vi "Teleop.vi"(10 "Match Info":T1={"Autonomous Elapsed Seconds"=0.0, "TeleOp Elapsed Seconds"=0.0, "Disabled Elapsed Seconds"=0.0, "Visited Autonomous"=FALSE, "Visited TeleOp"=FALSE, "Visited Disabled"=FALSE, "Autonomous Settings"={"Autonomous Style"=enum."Independent", "VI Refnum"=refnum}}, 11 "Call Context":T2) -> ()   [LabVIEW 2013]
doc: "This VI is called for each TeleOp packet received from the DS where the robot is not disabled. It is often used to read from the joysticks and update I/O or to update setpoints for timed control loops. It should complete and return within 20 milliseconds or it may miss DS packets."
uses:
  <vilib>/Rock Robotics/WPI/DriverStation/WPI_DriverStationDerivedRobotMode.ctl
  <vilib>/Rock Robotics/WPI/DriverStation/WPI_DriverStationMatch Info.ctl
  <vilib>/Rock Robotics/WPI/Relay/WPI_RelayValue.ctl
  Robot Global Data.vi
  <vilib>/Rock Robotics/WPI/RobotDrive/WPI_RobotDriveMecanumDrive_Cartesian.vi
  <vilib>/Rock Robotics/WPI/Joystick/WPI_JoystickGetSetRefNum.vi
  <vilib>/functionblocks/Edge Detection/Edge Detect/Edge Detect.vi
  <vilib>/Rock Robotics/WPI/RobotDrive/WPI_RobotDriveGetSetRefNum.vi
  <vilib>/functionblocks/FB Core/FB Core.xnode
  <vilib>/functionblocks/NI_FunctionBlock Libraries.lvlib
panel:
  in  "percent":dbl
  out "Loader Up":bool
  out "Right Trigger":bool
  out "Left Trigger":bool
  out "Loader Out":bool
  out "Ejector":bool
  out "Trigger":bool
  out "1 Cylinder":bool
  out "2 Cylinder":bool
  out "3 Cylinder":bool
  out "Motor Values":dbl[](array[numeric])
  out "Gyro Mode?":bool
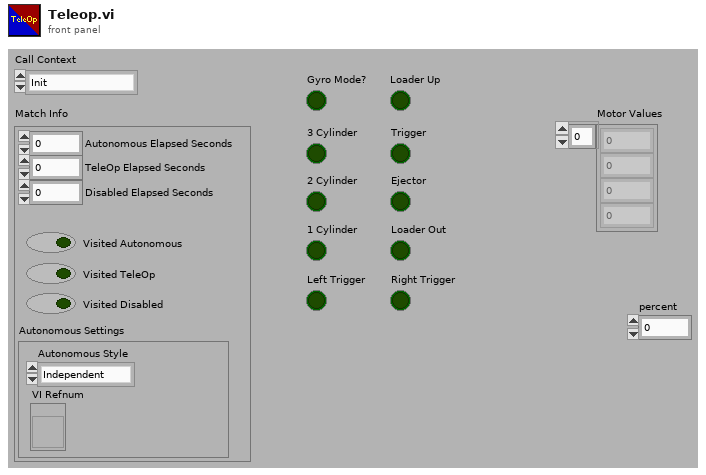
[diagram p1: front panel]
types:
  T1 = typedef "WPI_DriverStationMatch Info.ctl" = cluster{"Autonomous Elapsed Seconds":dbl, "TeleOp Elapsed Seconds":dbl, "Disabled Elapsed Seconds":dbl, "Visited Autonomous":bool, "Visited TeleOp":bool, "Visited Disabled":bool, "Autonomous Settings":cluster{"Autonomous Style":enum16{"Iterative", "Independent"}, "VI Refnum":refnum<vi>}}
  T2 = typedef "WPI_DriverStationDerivedRobotMode.ctl" = enum16{"Init", "Execute", "Stop"}
  T3 = typedef "WPI_RelayValue.ctl" = enum16{"Off", "On", "Forward", "Reverse"}
  T4 = typedef "WPI_MotorControlDeviceRef.ctl" = cluster{"DeviceStatus":errorcluster, "Type":enum16{"PWM", "CAN"}, "PWM":cluster{"Digital Module":T5, "PWM Channel":T6, "DeadBand":T7}, "CAN":cluster{"Device Number":u8, "Control Mode":T8, "Semaphore":T9, "Max Vout":dbl}, "Invert":bool, "TransformRef":T10, "InvTransformRef":T10}
  T5 = typedef "FPGA_TypedefDigitalModule.ctl" = enum16{"Digital Module 1", "Digital Module 2"}
  T6 = typedef "FPGA_DIOPWMChannel.ctl" = enum8{"PWM 1", "PWM 2", "PWM 3", "PWM 4", "PWM 5", "PWM 6", "PWM 7", "PWM 8", "PWM 9", "PWM 10", "Invalid"}
  T7 = typedef "WPI_PWMDeadband.ctl" = cluster{"Name":string, "maxPositivePwm":i32, "minPositivePwm":i32, "centerPwm":i32, "maxNegativePwm":i32, "minNegativePwm":i32, "angularRange":u16}
  T8 = typedef "WPI_CANJaguar_ControlMode.ctl" = enum8{"Percent VBus", "Current", "Speed", "Position", "Voltage"}
  T9 = typedef "Semaphore RefNum" = refnum<k1>
  T10 = typedef "WPI_PWMTransform_ConPane.ctl" = refnum<vi>
  T11 = typedef "WPI_JoystickDevRef.ctl" = cluster{"Device":T12}
  T12 = typedef "WPI_JoystickDeviceEnum.ctl" = enum16{"USB 1", "USB 2", "USB 3", "USB 4", "Kinect 1", "Kinect 2"}
  T13 = typedef "WPI_JoystickButtonState.ctl" = cluster{"Button 1":bool, "Button 2":bool, "Button 3":bool, "Button 4":bool, "Button 5":bool, "Button 6":bool, "Button 7":bool, "Button 8":bool, "Button 9":bool, "Button 10":bool, "Button 11":bool, "Button 12":bool}
  T14 = cluster{"axis 1 (x)":dbl, "axis 2 (y)":dbl, "axis 3 (throttle)":dbl, "axis 4":dbl, "axis 5":dbl, "axis 6":dbl}
  T15 = typedef "WPI_RelayDevRef.ctl" = cluster{"DevStatus":errorcluster, "Relay Channel":T16, "Digital Module":T5, "Relay Direction":T17}
  T16 = typedef "FPGA_DIORelayChannel.ctl" = enum8{"Relay 1", "Relay 2", "Relay 3", "Relay 4", "Relay 5", "Relay 6", "Relay 7", "Relay 8", "Invalid"}
  T17 = typedef "WPI_RelayDirection.ctl" = enum16{"Both directions", "Forward only", "Reverse only"}
  T18 = typedef "WPI_RobotDriveDevRef.ctl" = cluster{"DevStatus":errorcluster, "Motors[]":T4[], "Square Inputs":bool, "Max Output":dbl, "Isochronous":bool}
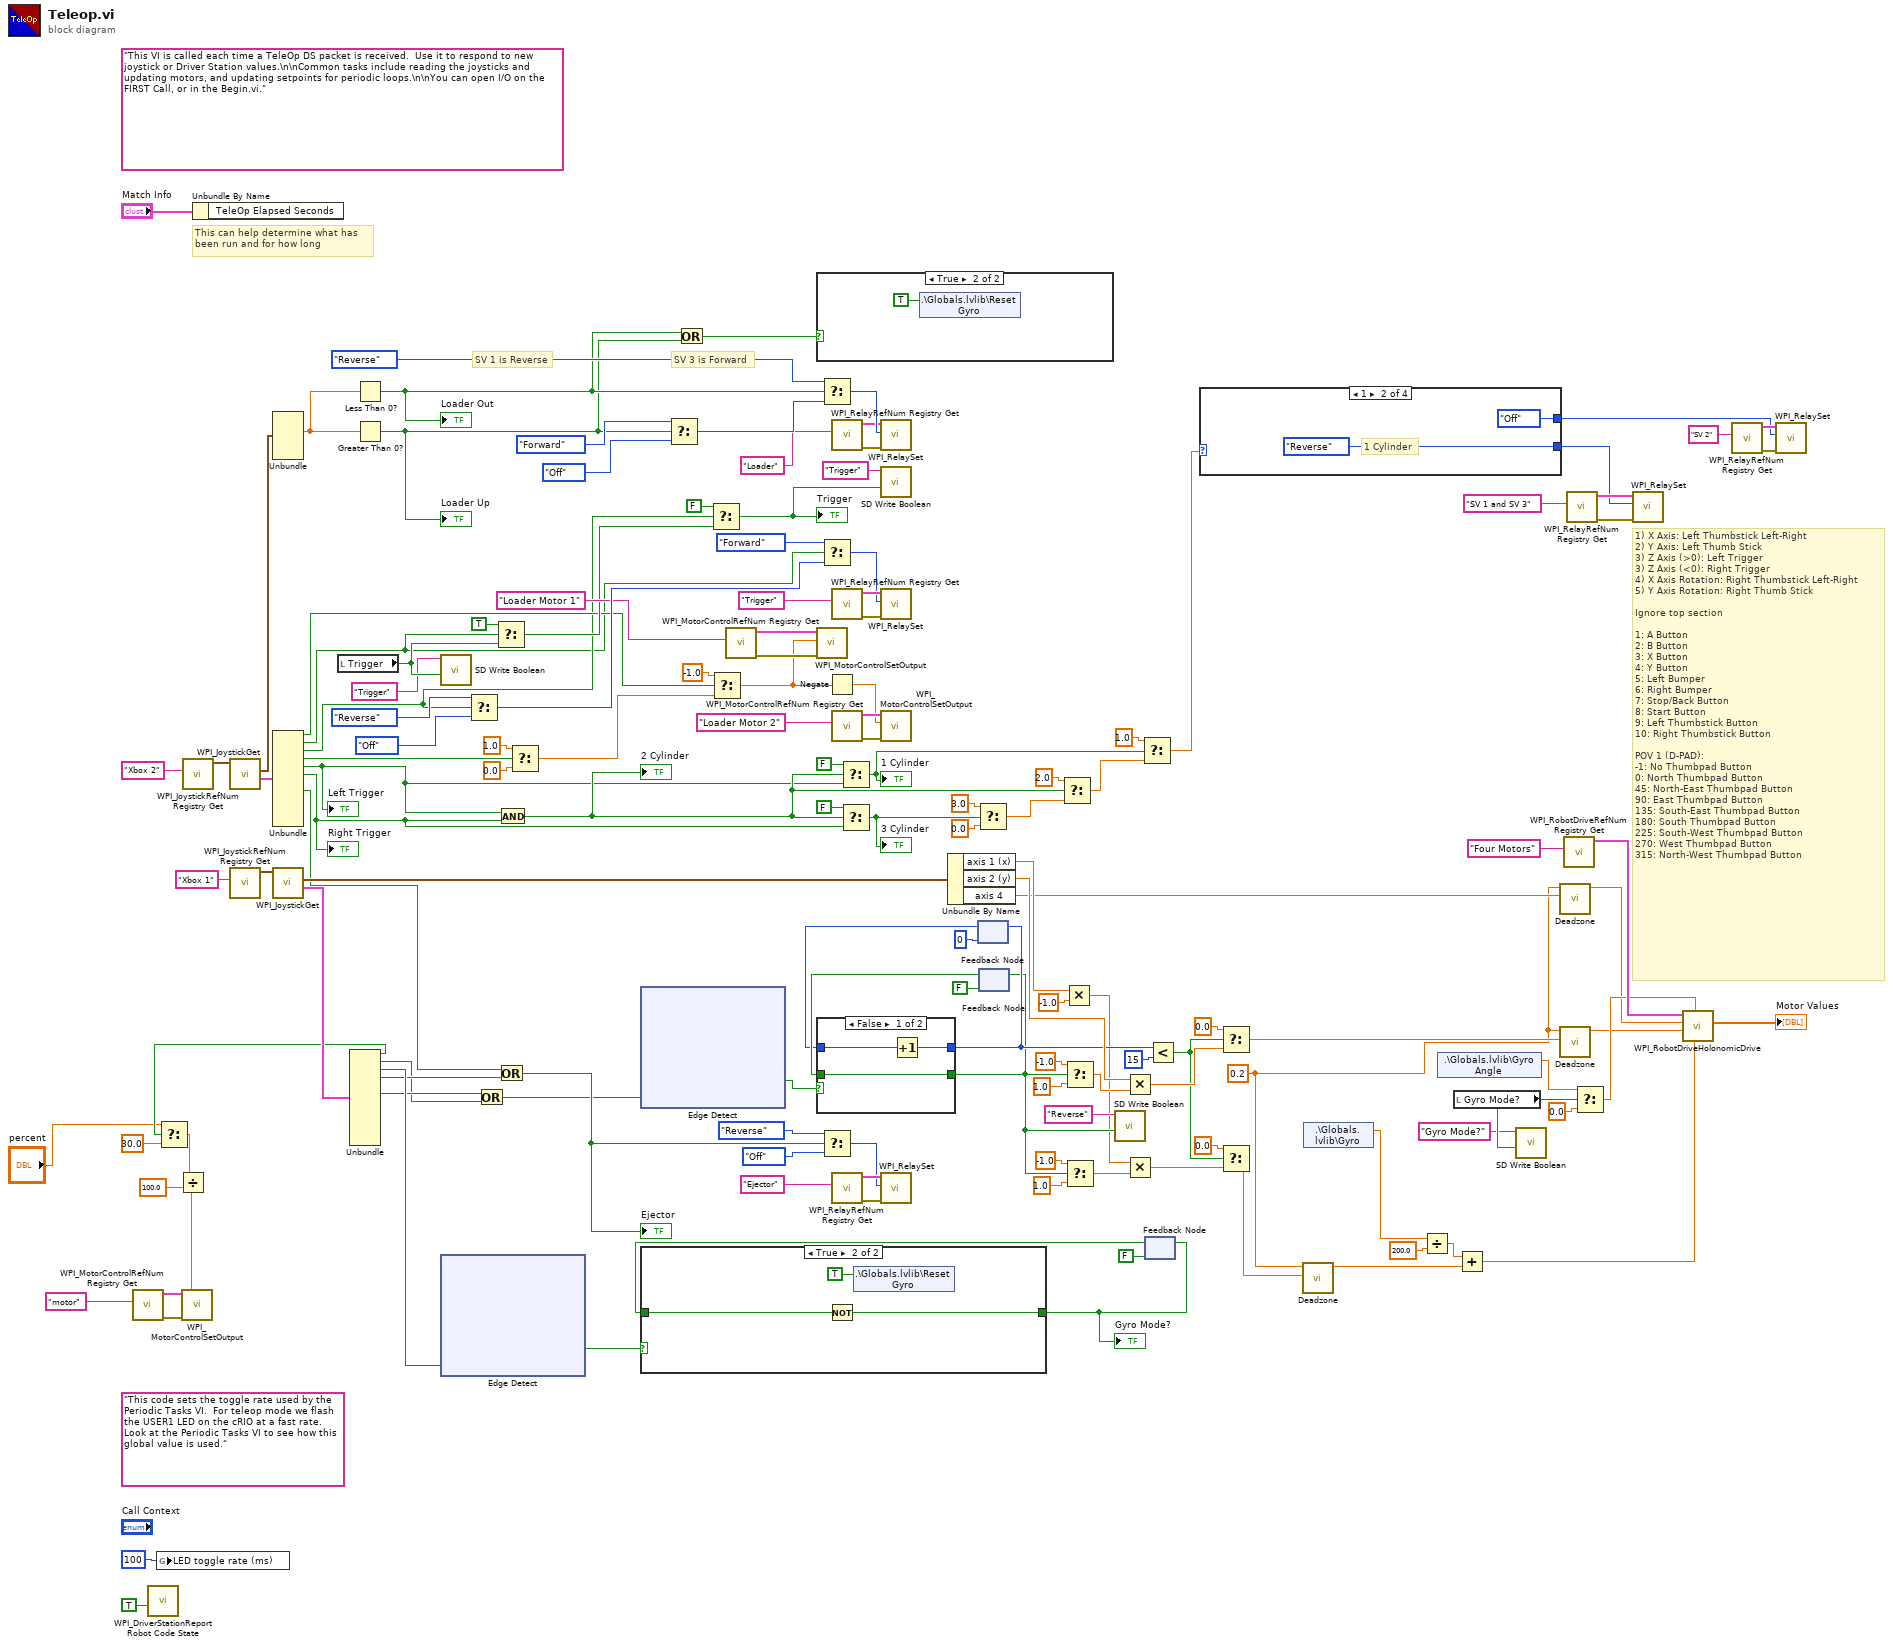
[diagram p0: block diagram]
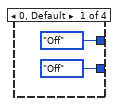
[diagram p3: hidden frame]
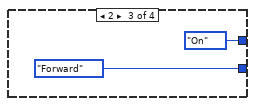
[diagram p4: hidden frame]
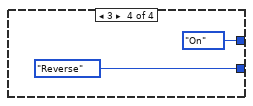
[diagram p5: hidden frame]
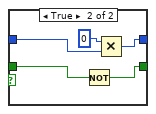
[diagram p6: hidden frame]
diagram:
  w19 = 0.2 ("Deadzone")
  (unwired) "This code sets the toggle rate used by the Periodic Tasks VI.  For teleop mode we flash the USER1 LED on the cRIO at a fast rate.  Look at the Periodic Tasks VI to see how this global value is used."
  (unwired) "This VI is called each time a TeleOp DS packet is received.  Use it to respond to new joystick or Driver Station values.\n\nCommon tasks include reading the joysticks and updating motors, and updating setpoints for periodic loops.\n\nYou can open I/O on the FIRST Call, or in the Begin.vi."
  # "SV 3 is Forward"
  # "SV 1 is Reverse"
  # "1) X Axis: Left Thumbstick Left-Right\n2) Y Axis: Left Thumb Stick\n3) Z Axis (>0): Left Trigger\n3) Z Axis (<0): Right Trigger\n4) X Axis Rotation: Right Thumbstick Left-Right\n5) Y Axis Rotation: Right Thumb Stick\n\nIgnore top section\n\n1: A Button\n2: B Button\n3: X Button\n4: Y Button\n5: Left Bumper\n6: Right Bumper\n7: Stop/Back Button\n8: Start Button\n9: Left Thumbstick Button\n10: Right Thumbstick Button\n\nPOV 1 (D-PAD):\n-1: No Thumbpad Button\n0: North Thumbpad Button\n45: North-East Thumbpad Button\n90: East Thumbpad Button\n135: South-East Thumbpad Button\n180: South Thumbpad Button\n225: South-West Thumbpad Button\n270: West Thumbpad Button\n315: North-West Thumbpad Button"
  # "This can help determine what has\nbeen run and for how long"
  n1 = call <vilib>:"WPI_MotorControlRefNum Registry Get.vi"("refnum name"="motor") -> ("error out"=w7:errorcluster, "MotorControlDevRef"=w8:T4)  [unwired: 9 in]
  n2 = call <vilib>:"WPI_DriverStationReport Robot Code State.vi"("TeleOp"=TRUE ("Autonomous")) -> ()  [unwired: 10 in, 1 out]
  n3 = global write "Robot Global Data.vi" "LED toggle rate (ms)"(u32 100 ("LED ms toggle rate")) -> ()
  n4 = call <vilib>:"WPI_JoystickRefNum Registry Get.vi"("refnum name"="Xbox 2") -> ("JoystickDevRef"=w112:T11)  [unwired: 1 in, 9 out]
  n5 = Unbundle By Name("Match Info") -> ()  [unwired: 1 out]
  n6 = call <vilib>:"WPI_JoystickGet.vi"("JoystickDevRef"=w112) -> ("Buttons"=w110:T13, "Axes"=w109:T14)  [unwired: 1 in, 4 out]
  n7 = call <vilib>:"WPI_JoystickRefNum Registry Get.vi"("refnum name"="Xbox 1") -> ("JoystickDevRef"=w143:T11)  [unwired: 1 in, 9 out]
  n8 = Unbundle(w109) -> ("axis 3 (throttle)"=w44:dbl)  [unwired: 5 out]
  n9 = Unbundle(w110) -> ("Button 1"=w32:bool, "Button 2"=w29:bool, "Button 3"=w30:bool, "Button 4"=w31:bool, "Button 5"=w45:bool, "Button 6"=w46:bool, "Button 8"=w35:bool)  [unwired: 5 out]
  "Left Trigger" <- w45
  "Right Trigger" <- w46
  n10 = call <vilib>:"WPI_JoystickGet.vi"("JoystickDevRef"=w143) -> ("Buttons"=w135:T13, "Axes"=w140:T14)  [unwired: 1 in, 4 out]
  n11 = local read "Trigger"() -> (w48:bool)
  n12 = Unbundle(w135) -> ("Button 1"=w6:bool, "Button 2"=w21:bool, "Button 3"=w49:bool, "Button 4"=w33:bool, "Button 6"=w22:bool)  [unwired: 7 out]
  n13 = Select(t="percent", s=w6, f=30.0) -> (s? t:f=w4:dbl)
  n14 = Divide(x=w4, y=100.0) -> (x/y=w2:dbl)
  n15 = call <vilib>:"WPI_MotorControlSetOutput.vi"("error in (no error)"=w7, "Output"=w2, "MotorControlDevRef"=w8) -> ()  [unwired: 6 in, 3 out]
  n16 = Less Than 0?(x=w44) -> (x < 0?=w17:bool)
  "Loader Out" <- w17
  n17 = Greater Than 0?(x=w44) -> (x > 0?=w16:bool)
  "Loader Up" <- w16
  n18 = call <vilib>:"SD Write Boolean.vi"("Boolean"=w48, "Name"="Trigger") -> ()  [unwired: 8 in, 2 out]
  n19 = xnode "Edge Detect"("input 1"=w49) -> ("output"=w53:bool)  [unwired: 2 in, 1 out]
  n20 = Select(t=WPI_RelayValue."Reverse" ("RelayValue"), s=w30, f=WPI_RelayValue."Off") -> (s? t:f=w91:T3)
  n21 = Or(x=w22, y=w21) -> (x .or. y?=w20:bool)
  n22 = Select(t=TRUE, s=w29, f=w48) -> (s? t:f=w60:bool)
  n23 = Or(x=w35, y=w33) -> (x .or. y?=w34:bool)
  "Ejector" <- w34
  n24 = And(x=w45, y=w46) -> (x .and. y?=w70:bool)
  "2 Cylinder" <- w70
  n25 = Select(t=1.0, s=w31, f=0.0) -> (s? t:f=w58:dbl)
  n26 = xnode "Edge Detect"("input 1"=w20) -> ("output"=w120:bool)  [unwired: 2 in, 1 out]
  n27 = Select(t=WPI_RelayValue."Forward" ("RelayValue"), s=w16, f=WPI_RelayValue."Off") -> (s? t:f=w86:T3)
  n28 = Or(x=w17, y=w16) -> (x .or. y?=w15:bool)
  n29 = Select(t=FALSE, s=w30, f=w60) -> (s? t:f=w27:bool)
  "Trigger" <- w27
  n30 = Select(t=-1.0, s=w32, f=w58) -> (s? t:f=w54:dbl)
  n31 = call <vilib>:"WPI_MotorControlRefNum Registry Get.vi"("refnum name"="Loader Motor 1") -> ("error out"=w64:errorcluster, "MotorControlDevRef"=w65:T4)  [unwired: 9 in]
  n32 = case shown="True" w15 {
    frame False {
    }
    frame True {
      n33 = shared-variable ".\\Globals.lvlib\\Reset Gyro"(TRUE ("Reset Gyro")) -> ()  [unwired: 1 in, 1 out]
    }
  }
  n34 = call <vilib>:"WPI_MotorControlSetOutput.vi"("error in (no error)"=w64, "Output"=w54, "MotorControlDevRef"=w65) -> ()  [unwired: 6 in, 3 out]
  n35 = Select(t=WPI_RelayValue."Reverse" ("RelayValue"), s=w17, f=w86) -> (s? t:f=w87:T3)
  n36 = Select(t=WPI_RelayValue."Forward" ("RelayValue"), s=w29, f=w91) -> (s? t:f=w90:T3)
  n37 = Select(t=WPI_RelayValue."Reverse" ("f"), s=w34, f=WPI_RelayValue."Off") -> (s? t:f=w72:T3)
  n38 = Negate(x=w54) -> (-x=w59:dbl)
  n39 = call <vilib>:"WPI_RelayRefNum Registry Get.vi"("refnum name"="Loader") -> ("error out"=w81:errorcluster, "RelayDevRef"=w82:T15)  [unwired: 9 in]
  n40 = call <vilib>:"WPI_RelayRefNum Registry Get.vi"("refnum name"="Trigger") -> ("error out"=w80:errorcluster, "RelayDevRef"=w95:T15)  [unwired: 9 in]
  n41 = call <vilib>:"WPI_MotorControlRefNum Registry Get.vi"("refnum name"="Loader Motor 2") -> ("error out"=w63:errorcluster, "MotorControlDevRef"=w66:T4)  [unwired: 9 in]
  n42 = call <vilib>:"WPI_RelayRefNum Registry Get.vi"("refnum name"="Ejector") -> ("error out"=w77:errorcluster, "RelayDevRef"=w75:T15)  [unwired: 9 in]
  n43 = Select(t=FALSE, s=w70, f=w45) -> (s? t:f=w71:bool)
  "1 Cylinder" <- w71
  n44 = Select(t=FALSE, s=w70, f=w46) -> (s? t:f=w69:bool)
  "3 Cylinder" <- w69
  n45 = call <vilib>:"WPI_RelaySet.vi"("error in (no error)"=w81, "RelayValue"=w87, "RelayDevRef"=w82) -> ()  [unwired: 7 in, 2 out]
  n46 = call <vilib>:"SD Write Boolean.vi"("Boolean"=w27, "Name"="Trigger") -> ()  [unwired: 8 in, 2 out]
  n47 = call <vilib>:"WPI_RelaySet.vi"("error in (no error)"=w80, "RelayValue"=w90, "RelayDevRef"=w95) -> ()  [unwired: 7 in, 2 out]
  n48 = call <vilib>:"WPI_MotorControlSetOutput.vi"("error in (no error)"=w63, "Output"=w59, "MotorControlDevRef"=w66) -> ()  [unwired: 6 in, 3 out]
  n49 = call <vilib>:"WPI_RelaySet.vi"("error in (no error)"=w77, "RelayValue"=w72, "RelayDevRef"=w75) -> ()  [unwired: 7 in, 2 out]
  n50 = Unbundle By Name(w140) -> ("axis 1 (x)"=w137:dbl, "axis 2 (y)"=w138:dbl, "axis 4"=w26:dbl)
  n51 = Select(t=3.0, s=w69, f=0.0) -> (s? t:f=w102:dbl)
  n52 = feedback #1(0) -> (w115:i32)
  n53 = feedback #2(FALSE) -> (w122:bool)
  n54 = case shown="False" w120 {
    tunnel: w122 -> [w149 w154]
    tunnel: [w149 w153] -> w37
    tunnel: w115 -> [w148 w152]
    tunnel: [w147 w150] -> w114
    frame False {
      n55 = Increment(x=w148) -> (x+1=w147:i32)
    }
    frame True {
      n56 = Not(x=w154) -> (.not. x?=w153:bool)
      n57 = Multiply(x=0, y=w152) -> (x*y=w150:i32)
    }
  }
  n58 = feedback-in #1(w114) -> ()
  n59 = feedback-in #2(w37) -> ()
  n60 = Select(t=2.0, s=w70, f=w102) -> (s? t:f=w100:dbl)
  n61 = Multiply(x=w137, y=-1.0) -> (x*y=w36:dbl)
  n62 = Select(t=-1.0, s=w37, f=1.0) -> (s? t:f=w125:dbl)
  n63 = Select(t=-1.0, s=w37, f=1.0) -> (s? t:f=w40:dbl)
  n64 = call <vilib>:"SD Write Boolean.vi"("Boolean"=w37, "Name"="Reverse") -> ()  [unwired: 8 in, 2 out]
  n65 = Multiply(x=w138, y=w125) -> (x*y=w118:dbl)
  n66 = Multiply(x=w36, y=w40) -> (x*y=w41:dbl)
  n67 = Select(t=1.0, s=w71, f=w100) -> (s? t:f=w98:dbl)
  n68 = feedback #3(FALSE) -> (w130:bool)
  n69 = case shown="True" w53 {
    tunnel: w130 -> [w155 w158]
    tunnel: [w155 w157] -> w128
    frame False {
    }
    frame True {
      n70 = Not(x=w158) -> (.not. x?=w157:bool)
      n71 = shared-variable ".\\Globals.lvlib\\Reset Gyro"(TRUE ("Reset Gyro")) -> ()  [unwired: 1 in, 1 out]
    }
  }
  "Gyro Mode?" <- w128
  n72 = feedback-in #3(w128) -> ()
  n73 = Less?(x=w114, y=15) -> (x < y?=w42:bool)
  n74 = case shown="1" w98 {
    tunnel: [WPI_RelayValue."Off" ("RelayValue") WPI_RelayValue."Reverse" ("RelayValue") WPI_RelayValue."Forward" ("RelayValue") WPI_RelayValue."Reverse" ("RelayValue")] -> w97
    tunnel: [WPI_RelayValue."Off" ("RelayValue") WPI_RelayValue."Off" ("RelayValue") WPI_RelayValue."On" ("RelayValue") WPI_RelayValue."On" ("RelayValue")] -> w96
    frame 0, Default {
    }
    frame 1 {
      # "1 Cylinder"
    }
    frame 2 {
    }
    frame 3 {
    }
  }
  n75 = Select(t=0.0, s=w42, f=w118) -> (s? t:f=w24:dbl)
  n76 = Select(t=0.0, s=w42, f=w41) -> (s? t:f=w25:dbl)
  n77 = call "Deadzone.vi"("Input"=w25, "Deadzone"=w19) -> ("Corected"=w12:dbl)  [unwired: 9 in]
  n78 = shared-variable ".\\Globals.lvlib\\Gyro"() -> (w10:dbl)  [unwired: 1 in, 1 out]
  n79 = Divide(x=w10, y=200.0) -> (x/y=w14:dbl)
  n80 = shared-variable ".\\Globals.lvlib\\Gyro Angle"() -> (w134:dbl)  [unwired: 1 in, 1 out]
  n81 = local read "Gyro Mode?"() -> (w132:bool)
  n82 = Add(x=w14, y=w12) -> (x+y=w11:dbl)
  n83 = call <vilib>:"SD Write Boolean.vi"("Boolean"=w132, "Name"="Gyro Mode?") -> ()  [unwired: 8 in, 2 out]
  n84 = call "Deadzone.vi"("Input"=w26, "Deadzone"=w19) -> ("Corected"=w18:dbl)  [unwired: 9 in]
  n85 = call "Deadzone.vi"("Input"=w24, "Deadzone"=w19) -> ("Corected"=w23:dbl)  [unwired: 9 in]
  n86 = call <vilib>:"WPI_RobotDriveRefNum Registry Get.vi"("refnum name"="Four Motors") -> ("RobotDriveDevRef"=w52:T18)  [unwired: 1 in, 9 out]
  n87 = call <vilib>:"WPI_RelayRefNum Registry Get.vi"("refnum name"="SV 1 and SV 3") -> ("error out"=w78:errorcluster, "RelayDevRef"=w126:T15)  [unwired: 9 in]
  n88 = Select(t=w134, s=w132, f=0.0) -> (s? t:f=w50:dbl)
  n89 = call <vilib>:"WPI_RelaySet.vi"("error in (no error)"=w78, "RelayValue"=w97, "RelayDevRef"=w126) -> ()  [unwired: 7 in, 2 out]
  n90 = call-poly <vilib>:"WPI_RobotDriveHolonomicDrive.vi"("Rotation"=w11, "Gyro Angle"=w50, "Y"=w23, "X"=w18, "RobotDriveDevRef"=w52) -> ("Motor Values"=→"Motor Values":dbl[])  [unwired: 4 in, 2 out]
  n91 = call <vilib>:"WPI_RelayRefNum Registry Get.vi"("refnum name"="SV 2") -> ("error out"=w79:errorcluster, "RelayDevRef"=w105:T15)  [unwired: 9 in]
  n92 = call <vilib>:"WPI_RelaySet.vi"("error in (no error)"=w79, "RelayValue"=w96, "RelayDevRef"=w105) -> ()  [unwired: 7 in, 2 out]
